vi "Write Frequencies.vi"(8 "error in (no error)":errorcluster, 10 "Frequencies":dbl[](array[numeric]), 11 "Write Frequencies Msg in":refnum<class "Write Frequencies Msg.lvclass">) -> (0 "error out":errorcluster, 3 "Write Frequencies Msg out":refnum<class "Write Frequencies Msg.lvclass">)   [LabVIEW 2015, in "Write Frequencies Msg.lvclass"]
uses:
  Write Frequencies Msg.lvclass
  Write Frequencies Msg.lvclass/Write Frequencies Msg.ctl
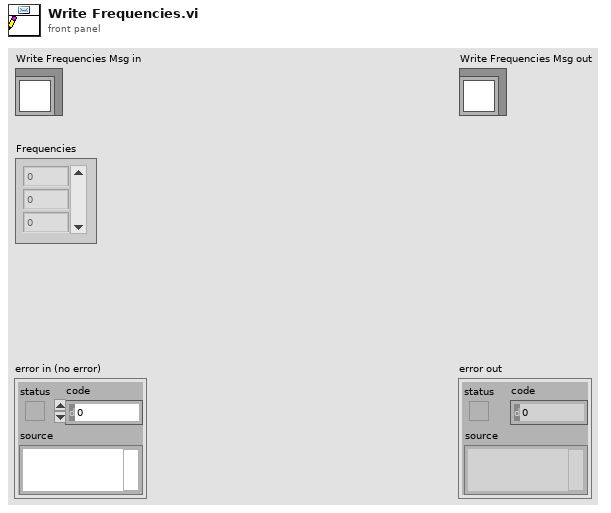
[diagram p1: front panel]
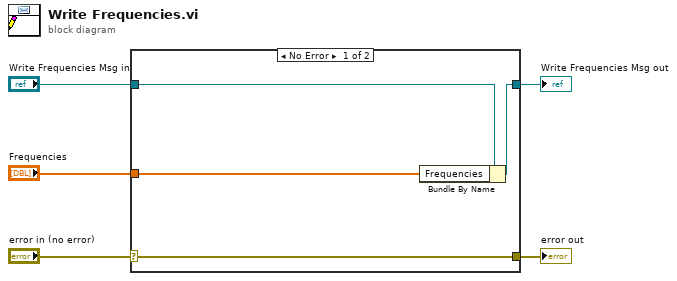
[diagram p0: block diagram]
diagram:
  n1 = case shown="No Error" "error in (no error)" {
    selector: "error in (no error)" -> [w9 w10]
    tunnel: [w9 w10] -> w4
    tunnel: [w7 w11] -> w2
    tunnel: "Write Frequencies Msg in" -> [w8 w11]
    tunnel: "Frequencies" -> [w6 _]
    frame No Error {
      n2 = Bundle By Name(cluster=w8, "Frequencies"=w6) -> (w7:refnum<class "Write Frequencies Msg.lvclass">)
    }
    frame Error {
    }
  }
  "error out" <- w4
  "Write Frequencies Msg out" <- w2
